vi "ERR_get_error.vi"(8 "error in (no error)":errorcluster, 11 "SSL-Lib in":refnum<class "SSL-Lib.lvclass">) -> (0 "error out":errorcluster, 3 "SSL-Lib out":refnum<class "SSL-Lib.lvclass">)   [LabVIEW 2013, in "OpenSSL Socket.lvlib" / "SSL-Lib.lvclass"]
uses:
  SSL-Lib.lvclass
  SSL-Lib.lvclass/SSL-Lib.ctl
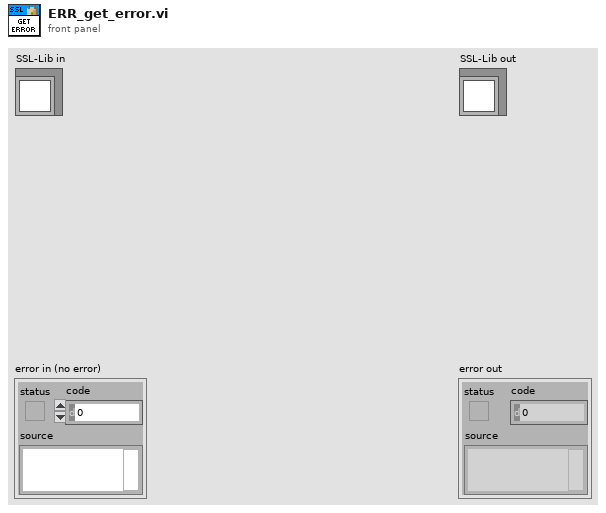
[diagram p1: front panel]
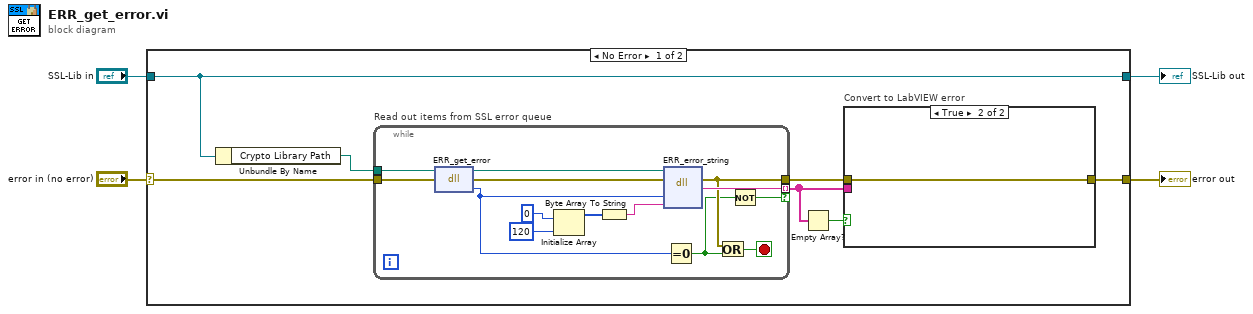
[diagram p0: block diagram]
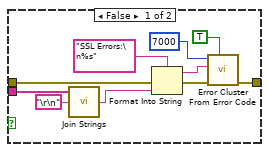
[diagram p2: hidden frame]
diagram:
  n1 = case shown="No Error" "error in (no error)" {
    selector: "error in (no error)" -> [w11 w38]
    tunnel: [w8 w38] -> w3
    tunnel: [w10 w37] -> w1
    tunnel: "SSL-Lib in" -> [w10 w37]
    frame No Error {
      n2 = Unbundle By Name(w10) -> ("Crypto Library Path"=w9:path)
      n3 = while "Read out items from SSL error queue" {
        tunnel: w9 -> [w35]
        tunnel: [w28] -> w5 mode=indexing if=w23
        tunnel: w11 -> [w36]
        tunnel: [w27] -> w6
        stop <- w26 stop-if-true
        n4 = dll-call lib="C:/Program Files (x86)/National Instruments/Shared/nissl/NIlibeay32.dll" fn="ERR_get_error"(path in=w35, error in=w36) -> (path out=w34:path, error out=w33:errorcluster, "return type"=w25:u32)  [unwired: 1 in]
        n5 = Initialize Array(u8 0, 120 ("dimension size")) -> (w30:u8[])
        n6 = Byte Array To String(unsigned byte array=w30) -> (string=w29:string)
        n7 = dll-call lib="C:/Program Files (x86)/National Instruments/Shared/nissl/NIlibeay32.dll" fn="ERR_error_string"(path in=w34, error in=w33, "e"=w25, "buf"=w29) -> (error out=w27:errorcluster, "return type"=w28:string)  [unwired: 3 in, 1 out]
        n8 = Equal To 0?(x=w25) -> (x = 0?=w24:bool)
        n9 = Or(x=w27, y=w24) -> (x .or. y?=w26:bool)
        n10 = Not(x=w24) -> (.not. x?=w23:bool)
      }
      n11 = Empty Array?(array=w5) -> (empty?=w7:bool)
      n12 = case "Convert to LabVIEW error" shown="True" w7 {
        tunnel: [w21 w22] -> w8
        tunnel: w6 -> [w17 w22]
        tunnel: w5 -> [w19 _]
        frame False {
          n13 = call <vilib>:"Join Strings.vi"("Separator (,)"="\r\n", "Strings In"=w19) -> ("String"=w14:string)  [unwired: 1 in]
          n14 = Format Into String(format string="SSL Errors:\n%s", error in=w17, w14) -> (resulting string=w15:string, error out=w16:errorcluster)  [unwired: 1 in]
          n15 = call <vilib>:"Error Cluster From Error Code.vi"("show call chain? (False)"=TRUE, "error in (no error)"=w16, "error message (\"\")"=w15, "error code (0)"=7000) -> ("error out"=w21:errorcluster)  [unwired: 5 in]
        }
        frame True {
        }
      }
    }
    frame Error {
    }
  }
  "error out" <- w3
  "SSL-Lib out" <- w1
